vi "GEOM_Adjust1DetReadMode.vi"(8 "GEOM_BinCorrectedFPA":T1, 9 "detectors":T2[](array[typedef]), 10 "Amplifiers":T3[](array[typedef]) {"fliped" items=["none", "horizontal", "vertical"]; "type" items=["LL", "LR", "UL", "UR"]}) -> (1 "detectors out":T2[](array[typedef]))   [LabVIEW 2016]
uses:
  GEOM_Amplifier.ctl
  GEOM_AmpType.ctl
  GEOM_ROI.ctl
  GEOM_Coords.ctl
  GEOM_DetSummaryStruct.ctl
  GEOM_CorrectedFPA.ctl
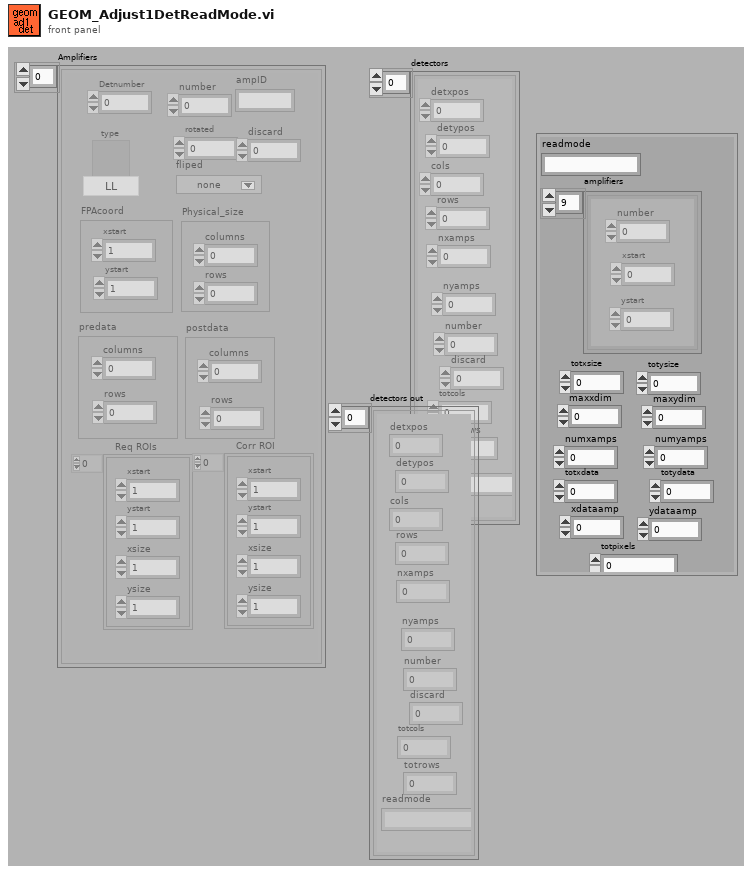
[diagram p1: front panel]
types:
  T1 = typedef "GEOM_CorrectedFPA.ctl" = cluster{"readmode":string, "amplifiers":cluster{"number":i32, "xstart":i32, "ystart":i32}[], "totxsize":i32, "totysize":i32, "maxxdim":i32, "maxydim":i32, "numxamps":i32, "numyamps":i32, "totxdata":i32, "totydata":i32, "xdataamp":i32, "ydataamp":i32, "totpixels":i32}
  T2 = typedef "GEOM_DetSummaryStruct.ctl" = cluster{"detxpos":i32, "detypos":i32, "cols":i32, "rows":i32, "nxamps":i32, "nyamps":i32, "number":i32, "discard":i32, "totcols":i32, "totrows":i32, "readmode":string}
  T3 = typedef "GEOM_Amplifier.ctl" = cluster{"number":i32, "type":T4, "rotated":i16, "fliped":u16, "FPAcoord":cluster{"xstart":i32, "ystart":i32}, "Physical_size":cluster{"columns":i32, "rows":i32}, "predata":cluster{"columns":i32, "rows":i32}, "postdata":cluster{"columns":i32, "rows":i32}, "Req ROIs":T5, "Corr ROI":T5, "Detnumber":i32, "ampID":string, "discard":i32}
  T4 = typedef "GEOM_AmpType.ctl" = u16
  T5 = typedef "GEOM_ROI.ctl" = T6[]
  T6 = typedef "GEOM_Coords.ctl" = cluster{"xstart":u32, "ystart":u32, "xsize":u32, "ysize":u32}
  T7 = cluster{"number":i32, "xstart":i32, "ystart":i32}[]
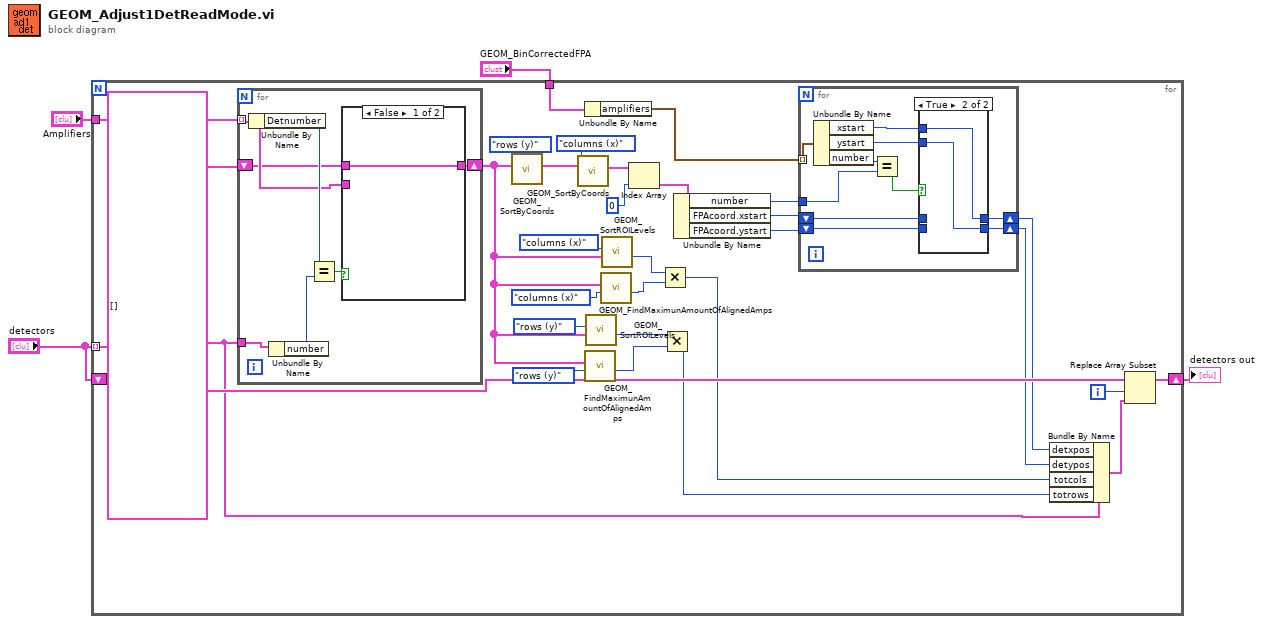
[diagram p0: block diagram]
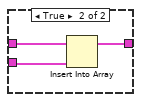
[diagram p3: hidden frame]
diagram:
  n1 = for {
    tunnel: "detectors" -> [w28] mode=indexing
    tunnel: "Amplifiers" -> [w35]
    shift-right: [w26] -> w2
    shift-left: "detectors" -> [w29]
    tunnel: "GEOM_BinCorrectedFPA" -> [w12]
    i -> [w13]
    n2 = for {
      tunnel: w35 -> [w52] mode=indexing
      tunnel: w28 -> [w55]
      shift-right: [w50] -> w20
      shift-left: T3[] [] -> [w51]
      n3 = Unbundle By Name(w52) -> ("Detnumber"=w56:i32)
      n4 = Unbundle By Name(w55) -> ("number"=w54:i32)
      n5 = Equal?(x=w56, y=w54) -> (x = y?=w53:bool)
      n6 = case shown="False" w53 {
        tunnel: w52 -> [_ w59]
        tunnel: [w57 w58] -> w50
        tunnel: w51 -> [w57 w60]
        frame False {
        }
        frame True {
          n7 = Insert Into Array(array=w60, new element=w59) -> (w58:T3[])  [unwired: 1 in]
        }
      }
    }
    n8 = call "GEOM_SortByCoords.vi"("amplifiers"=w20, "how"=enum16{"rows (y)", "columns (x)"}."rows (y)") -> ("sorted amplifiers"=w32:T3[])  [unwired: 9 out]
    n9 = call "GEOM_SortByCoords.vi"("amplifiers"=w32, "how"=enum16{"rows (y)", "columns (x)"}."columns (x)") -> ("sorted amplifiers"=w25:T3[])  [unwired: 9 out]
    n10 = Unbundle By Name(w12) -> ("amplifiers"=w11:T7)
    n11 = call "GEOM_FindMaximunAmountOfAlignedAmps.vi"("how"=enum16{"rows (y)", "columns (x)"}."rows (y)", "amplifiers"=w20) -> ("maxalignedamps"=w15:i32)  [unwired: 9 out]
    n12 = call "GEOM_SortROILevels.vi"("amplifiers"=w20, "how"=enum16{"rows (y)", "columns (x)"}."rows (y)") -> ("totpix"=w16:u32)  [unwired: 2 in, 7 out]
    n13 = call "GEOM_FindMaximunAmountOfAlignedAmps.vi"("how"=enum16{"rows (y)", "columns (x)"}."columns (x)", "amplifiers"=w20) -> ("maxalignedamps"=w18:i32)  [unwired: 9 out]
    n14 = call "GEOM_SortROILevels.vi"("amplifiers"=w20, "how"=enum16{"rows (y)", "columns (x)"}."columns (x)") -> ("totpix"=w19:u32)  [unwired: 2 in, 7 out]
    n15 = Index Array(array=w25, index=0) -> (element=w10:T3)
    n16 = Multiply(x=w19, y=w18) -> (x*y=w17:u32)
    n17 = Multiply(x=w16, y=w15) -> (x*y=w14:u32)
    n18 = Unbundle By Name(w10) -> ("number"=w7:i32, "FPAcoord.xstart"=w9:i32, "FPAcoord.ystart"=w8:i32)
    n19 = for {
      tunnel: w11 -> [w45] mode=indexing
      shift-right: [w39] -> w5
      shift-left: w8 -> [w36]
      shift-right: [w41] -> w6
      shift-left: w9 -> [w37]
      tunnel: w7 -> [w42]
      n20 = Unbundle By Name(w45) -> ("xstart"=w40:i32, "ystart"=w38:i32, "number"=w44:i32)
      n21 = Equal?(x=w44, y=w42) -> (x = y?=w43:bool)
      n22 = case shown="True" w43 {
        tunnel: [w47 w49] -> w41
        tunnel: w40 -> [_ w49]
        tunnel: [w46 w48] -> w39
        tunnel: w38 -> [_ w48]
        tunnel: w37 -> [w47 _]
        tunnel: w36 -> [w46 _]
        frame False {
        }
        frame True {
        }
      }
    }
    n23 = Bundle By Name(cluster=w28, "detxpos"=w6, "detypos"=w5, "totcols"=w17, "totrows"=w14) -> (w27:T2)
    n24 = Replace Array Subset(array=w29, new element=w27, index=w13) -> (w26:T2[])
  }
  "detectors out" <- w2
